vi "LDP Control.vi"() -> ()   [LabVIEW 2017]
uses:
  <instrlib>/tio-labview/TIO Library/TIO Stream Open.vi
  <instrlib>/tio-labview/TIO Library/TIO RPC Send REQuest.vi
  <vilib>/Utility/error.llb/Clear Errors.vi
  <instrlib>/tio-labview/TIO Library/TIO RPC Parse Reply.vi
  <instrlib>/tio-labview/TIO Library/TIO RPC Parse Reply Error.vi
  <instrlib>/tio-labview/TIO Library/TIO Data Stream Parse timebase Info.vi
  <instrlib>/tio-labview/TIO Library/TIO Data Stream Parse pstream Info.vi
  <instrlib>/tio-labview/TIO Library/TIO Data Stream Parse dstream Info.vi
  <vilib>/Utility/High Resolution Relative Seconds.vi
  <instrlib>/tio-labview/TIO Library/TIO Serial Port Name Search.vi
  <instrlib>/tio-labview/TIO Library/TIO Stream Write.vi
  <instrlib>/tio-labview/TIO Library/TIO RPC Form Request.vi
  <instrlib>/tio-labview/TIO Library/TIO SLIP Serial Write.vi
  <instrlib>/tio-labview/TIO Library/TIO Form Packet.vi
  <instrlib>/tio-labview/TIO Library/TIO SLIP Encode.vi
  <instrlib>/tio-labview/TIO Library/TIO Serial Checksum CRC32.vi
  <vilib>/Utility/tcp.llb/UDP Multicast Open.vi
  <vilib>/Utility/tcp.llb/UDP Multicast Read-Write Open.vi
  <instrlib>/tio-labview/TIO Library/TIO Serial Port Discovery.vi
  <vilib>/Instr/_visa.llb/VISA Configure Serial Port (Instr).vi
  <instrlib>/tio-labview/TIO Library/TIO RPC Blocking.vi
  <instrlib>/tio-labview/TIO Library/TIO Stream Read Non-blocking.vi
  <instrlib>/tio-labview/TIO Library/TIO RPC Send Heartbeat.vi
panel:
  in  "Pulse rate":dbl[unit] format="%#_4g"
  in  "Cal Temperature":dbl[unit] format="%#_4g"
  in  "Laser Voltage":dbl[unit] format="%#_4g"
  out "Resistance":dbl[unit] format="%#_4g"
  in  "Calibrate R0":bool
  in  "TEC Enable":bool
  out "Temperature":dbl[unit] format="%#_4g"
  in  "Temperature Set":dbl[unit] format="%#_4g"
  in  "URL":refnum<visa-resource-name>="tcp://localhost"
  out "ID":string
  in  "Quit":bool
  in  "Duration":dbl[unit]=100.0
  in  "Reset":bool
  out "Temperature Graph":T1(graph)
  # "Pulsed Laser"
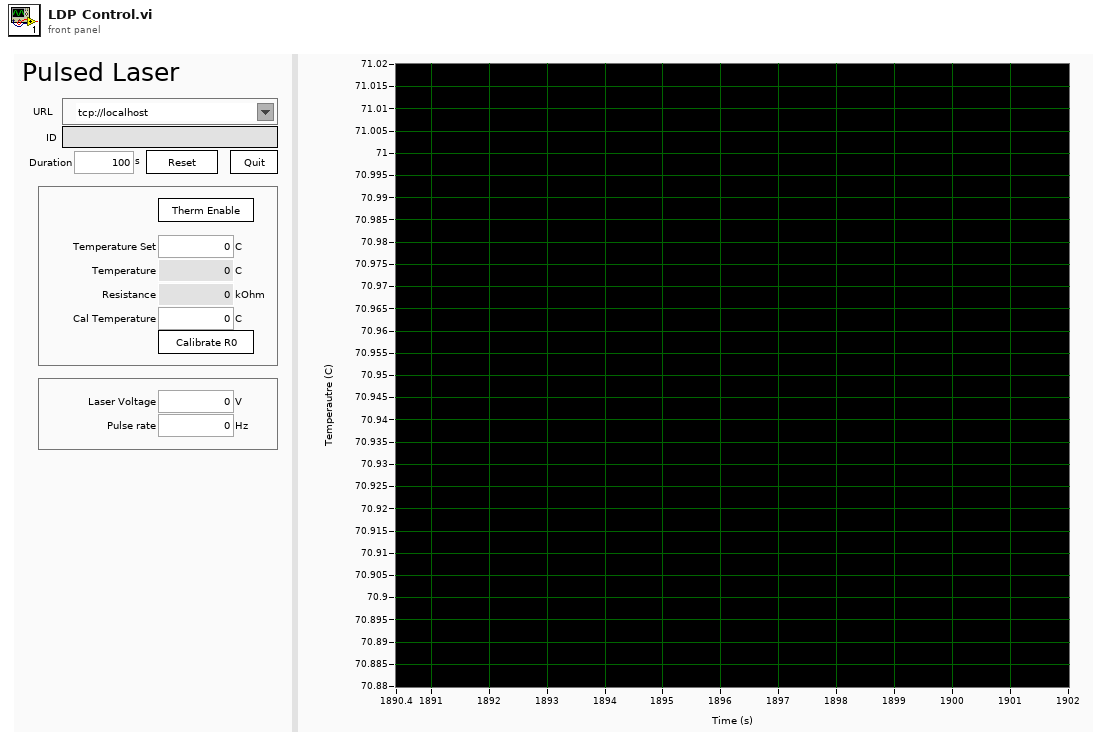
[diagram p1: front panel]
types:
  T1 = cluster{"start":dbl, "dt":dbl, "Timeseries":dbl[]}
  T2 = cluster{"TS Connection":cluster{"Type":enum16{"Serial", "TCP", "UDP", "mUDP"}, "URL":refnum<visa-resource-name>, "TO":u32, "Addr":u32, "Port":i32, "TCP":refnum<k5>, "UDP":refnum<k16>, "Route":string}, "REQ":refnum<queue>, "REP":refnum<queue>}
  T3 = cluster{"Awaiting REP":bool, "REQ ID":u32, "streams in":cluster{"id":u16, "timebase id":u16, "period":u32, "offset":u32, "sample number":u64, "total components":u16, "flags":u16, "components":cluster{"source id":u16, "flags":u16, "period":u32, "offset":u32}[]}[], "sources":cluster{"id":u16, "timebase_id":u16, "period":u32, "offset":u32, "fmt":i32, "flags":u16, "channels":u16, "type":u8, "name":string, "column names":string[], "title":string, "units":string}[], "timebases":cluster{"id":u16, "source":u8, "epoch":u8, "start time":u64, "period numerator (µs)":u32, "period denominator (µs)":u32, "flags":u32, "stability":sgl, "source id":string}[]}
  T4 = cluster{"stream ID":u16, "Sample Number":u32, "Raw Data":string}
  T5 = cluster{"TC Connection":cluster{"Type":enum16{"Serial", "TCP", "UDP", "mUDP"}, "URL":refnum<visa-resource-name>, "TO":u32, "Addr":u32, "Port":i32, "TCP":refnum<k5>, "UDP":refnum<k16>, "Route":string}, "REQ":refnum<queue>, "REP":refnum<queue>}
  T6 = cluster{"Name":string, "Waveform":cluster{"start":dbl, "dt":dbl, "Timeseries":dbl[][]}}[]
  T7 = cluster{"start":dbl, "dt":dbl, "Timeseries":dbl[][]}
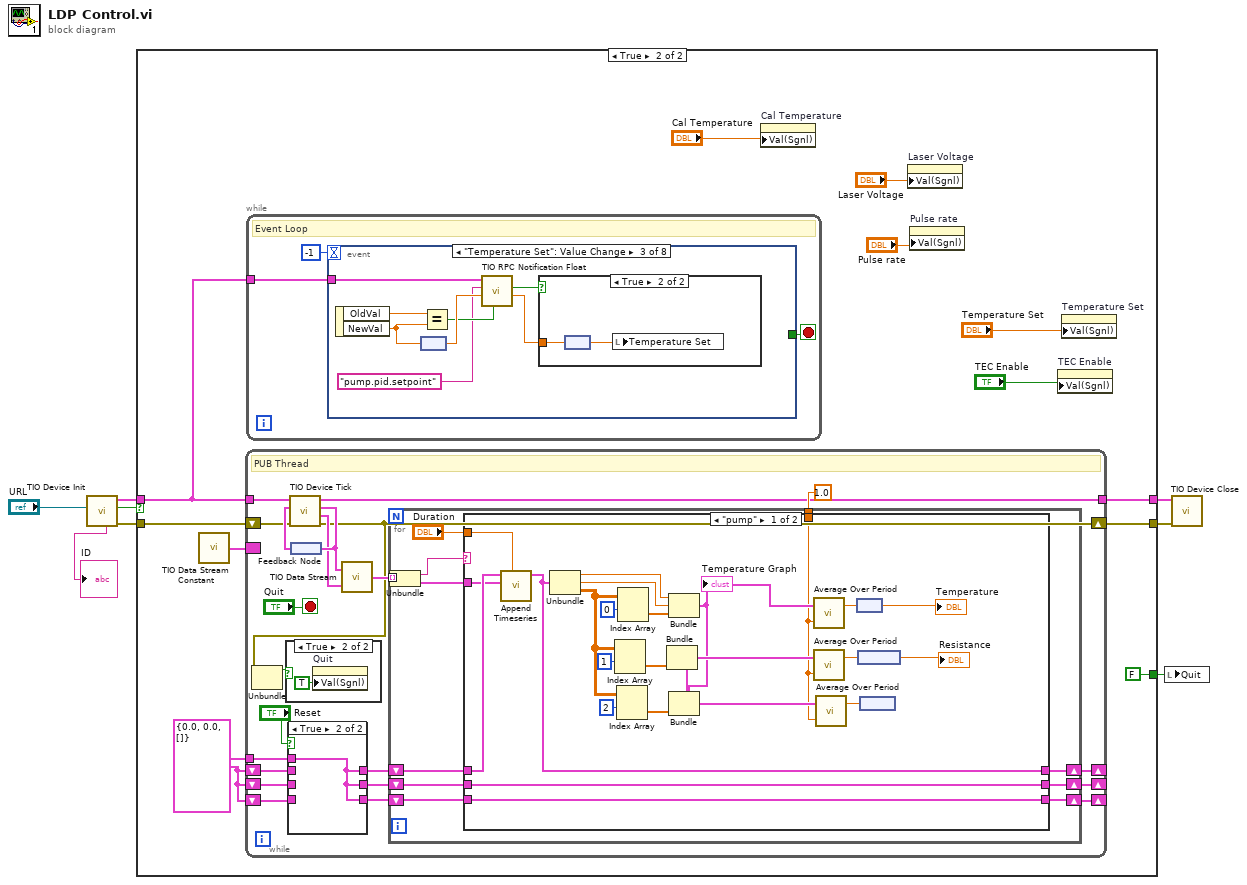
[diagram p0: block diagram]
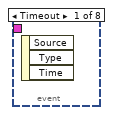
[diagram p6: hidden frame]
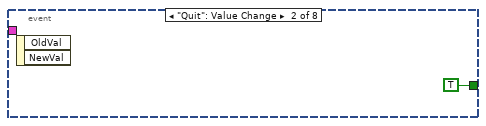
[diagram p7: hidden frame]
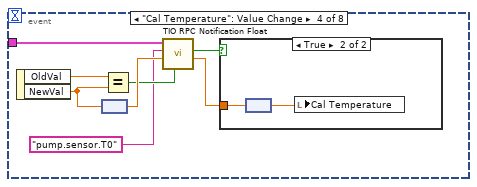
[diagram p9: hidden frame]
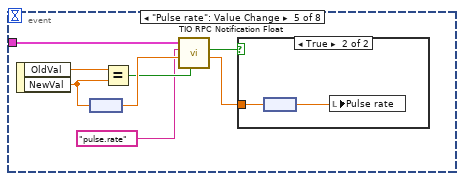
[diagram p11: hidden frame]
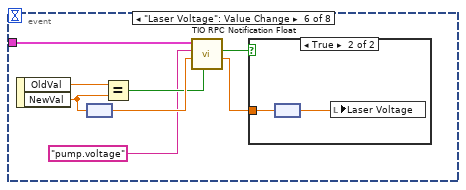
[diagram p13: hidden frame]
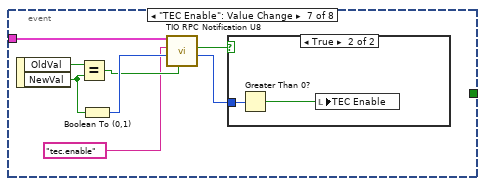
[diagram p15: hidden frame]
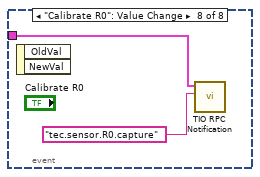
[diagram p17: hidden frame]
diagram:
  n1 = call <instrlib>:"TIO Device Init.vi"("URL"="URL") -> ("error out"=w5:errorcluster, 2:"ID Verified"=w6:bool, "TIO"=w7:T2, 4:"ID Verified"=→"ID":string)  [unwired: 6 in, 1 out]
  n2 = case shown="True" w6 {
    tunnel: w7 -> [w10 w17]
    tunnel: w5 -> [w9 w18]
    tunnel: [_ FALSE ("Quit")] -> w4
    tunnel: [w9 w13] -> w3
    tunnel: [w10 w12] -> w2
    frame False {
    }
    frame True {
      w14 = cluster{dbl, dbl, dbl[][]} {0.0, 0.0, []} ("Waveform Timeseries")
      n3 = call <instrlib>:"TIO Data Stream Constant.vi"() -> ("TIO State"=w19:T3)
      n4 = while {
        shift-right: [w44] -> _
        shift-left: w14 -> [w34]
        border: w19 -> [_]
        tunnel: w17 -> [w40]
        tunnel: w14 -> [w33]
        shift-right: [w31] -> _
        shift-left: w14 -> [w30]
        shift-right: [w27] -> _
        shift-left: w14 -> [w28]
        tunnel: [w24] -> w12
        shift-right: [w23] -> w13
        shift-left: w18 -> [w39]
        stop <- "Quit" stop-if-true
        # "PUB Thread"
        n5 = case shown="True" "Reset" {
          tunnel: [w48 w49] -> w35
          tunnel: w34 -> [w48 _]
          tunnel: w33 -> [_ w49]
          tunnel: [w47 w49] -> w32
          tunnel: w30 -> [w47 _]
          tunnel: w28 -> [w46 _]
          tunnel: [w46 w49] -> w29
          frame False {
          }
          frame True {
          }
        }
        n6 = feedback #1() -> (w43:T3)
        n7 = call <instrlib>:"TIO Device Tick.vi"("Error in"=w39, "TIO State"=w43, "TIO"=w40) -> ("Error out"=w23:errorcluster, "Data Out"=w41:T4, "TIO State"=w42:T3, "TIO"=w24:T5)  [unwired: 5 in]
        n8 = Unbundle(w23) -> ("status"=w25:bool)  [unwired: 2 out]
        n9 = case shown="True" w25 {
          frame False {
          }
          frame True {
            n10 = property on="Quit" class="Bool (strict)"("Val(Sgnl)"=TRUE ("Value (Signaling)")) -> ()  [unwired: 2 in, 2 out]
          }
        }
        n11 = feedback-in #1(w42) -> ()
        n12 = call <instrlib>:"TIO Data Stream.vi"("Raw Data"=w41, "TIO State"=w42) -> ("Data Out"=w38:T6)
        n13 = for {
          shift-right: [w59] -> w44
          shift-left: w35 -> [w58]
          tunnel: w38 -> [w57] mode=indexing
          shift-right: [w53] -> w31
          shift-left: w32 -> [w54]
          shift-right: [w51] -> w27
          shift-left: w29 -> [w52]
          tunnel: dbl[unit] 1.0 ("Period") -> [w50]
          n14 = Unbundle(w57) -> ("Name"=w55:string, "Waveform"=w56:T7)
          n15 = case shown="\"pump\"" w55 {
            tunnel: "Duration" -> [w84 _]
            tunnel: [w82 w87] -> w59
            tunnel: w58 -> [w81 w87]
            tunnel: w56 -> [w64 _]
            tunnel: w54 -> [w63 w86]
            tunnel: [w63 w86] -> w53
            tunnel: [w62 w85] -> w51
            tunnel: w52 -> [w62 w85]
            tunnel: w50 -> [w61 _]
            frame "pump" {
              n16 = call <instrlib>:"Append Timeseries.vi"("Duration"=w84, "In New"=w64, "In Old"=w81) -> ("Appended"=w82:T7)  [unwired: 8 in]
              n17 = Unbundle(w82) -> ("start"=w68:dbl, "dt"=w67:dbl, "Timeseries"=w69:dbl[][])
              n18 = Index Array(array=w69, index (row)=1 ("disabled index (col)")) -> (element=w71:dbl[])  [unwired: 1 in]
              n19 = Index Array(array=w69, index (row)=2 ("disabled index (col)")) -> (element=w76:dbl[])  [unwired: 1 in]
              n20 = Index Array(array=w69, index (row)=0 ("disabled index (col)")) -> (element=w80:dbl[])  [unwired: 1 in]
              n21 = Bundle("start"=w68, "dt"=w67, "Timeseries"=w80) -> (w65:T1)  [unwired: 1 in]
              "Temperature Graph" <- w65
              n22 = Bundle(cluster=w65, "Timeseries"=w71) -> (w72:T1)  [unwired: 2 in]
              n23 = Bundle(cluster=w65, "Timeseries"=w76) -> (w75:T1)  [unwired: 2 in]
              n24 = call <instrlib>:"Average Over Period.vi"("Average Period"=w61, "Waveform"=w65) -> ("Average"=w79:dbl)  [unwired: 1 in]
              n25 = call <instrlib>:"Average Over Period.vi"("Average Period"=w61, "Waveform"=w72) -> ("Average"=w73:dbl)  [unwired: 1 in]
              n26 = call <instrlib>:"Average Over Period.vi"("Average Period"=w61, "Waveform"=w75) -> ("Average"=w74:dbl)  [unwired: 1 in]
              n27 = node(w79) -> (→"Temperature":dbl[unit])
              n28 = node(w73) -> (→"Resistance":dbl[unit])
              n29 = node(w74) -> ()  [unwired: 1 out]
            }
            frame Default {
            }
          }
        }
      }
      n30 = while {
        tunnel: w17 -> [w89]
        stop <- w88 stop-if-true
        # "Event Loop"
        n31 = event shown="[2] \"Temperature Set\": Value Change" {
          selector: _ -> [_ _ _ _ _ _ _ _]
          dyn-events: _ -> [_ _ _ _ _ _ _ _]
          timeout: -1 -> [_ _ _ _ _ _ _ _]
          tunnel: w89 -> [_ _ w94 w104 w114 w124 w134 w143]
          tunnel: [_ TRUE ("Quit") _ _ _ _ _ _] -> w88
          event Timeout {
            n32 = event-data() -> ()  [unwired: 1 in, 3 out]
          }
          event "Quit": Value Change {
            n33 = event-data() -> ()  [unwired: 1 in, 2 out]
          }
          event "Temperature Set": Value Change {
            n34 = event-data() -> ("OldVal"=w99:dbl[unit], "NewVal"=w95:dbl[unit])  [unwired: 1 in]
            n35 = node(w95) -> (w98:dbl)
            n36 = Equal?(x=w99, y=w95) -> (x = y?=w93:bool)
            n37 = call <instrlib>:"TIO RPC Notification Float.vi"("Read"=w93, "Set value"=w98, "Topic"="pump.pid.setpoint" ("String"), "TIO"=w94) -> ("Get value (default if error)"=w96:sgl, "Response"=w97:bool)  [unwired: 4 in, 1 out]
            n38 = case shown="True" w97 {
              tunnel: w96 -> [_ w101]
              frame False {
              }
              frame True {
                n39 = node(w101) -> (w100:sgl[unit])
                n40 = local write "Temperature Set"(w100) -> ()
              }
            }
          }
          event "Cal Temperature": Value Change {
            n41 = event-data() -> ("OldVal"=w109:dbl[unit], "NewVal"=w105:dbl[unit])  [unwired: 1 in]
            n42 = node(w105) -> (w108:dbl)
            n43 = Equal?(x=w109, y=w105) -> (x = y?=w103:bool)
            n44 = call <instrlib>:"TIO RPC Notification Float.vi"("Read"=w103, "Set value"=w108, "Topic"="pump.sensor.T0" ("String"), "TIO"=w104) -> ("Get value (default if error)"=w106:sgl, "Response"=w107:bool)  [unwired: 4 in, 1 out]
            n45 = case shown="True" w107 {
              tunnel: w106 -> [_ w111]
              frame False {
              }
              frame True {
                n46 = node(w111) -> (w110:sgl[unit])
                n47 = local write "Cal Temperature"(w110) -> ()
              }
            }
          }
          event "Pulse rate": Value Change {
            n48 = event-data() -> ("OldVal"=w119:dbl[unit], "NewVal"=w115:dbl[unit])  [unwired: 1 in]
            n49 = node(w115) -> (w118:dbl)
            n50 = Equal?(x=w119, y=w115) -> (x = y?=w113:bool)
            n51 = call <instrlib>:"TIO RPC Notification Float.vi"("Read"=w113, "Set value"=w118, "Topic"="pulse.rate" ("String"), "TIO"=w114) -> ("Get value (default if error)"=w116:sgl, "Response"=w117:bool)  [unwired: 4 in, 1 out]
            n52 = case shown="True" w117 {
              tunnel: w116 -> [_ w121]
              frame False {
              }
              frame True {
                n53 = node(w121) -> (w120:sgl[unit])
                n54 = local write "Pulse rate"(w120) -> ()
              }
            }
          }
          event "Laser Voltage": Value Change {
            n55 = event-data() -> ("OldVal"=w129:dbl[unit], "NewVal"=w125:dbl[unit])  [unwired: 1 in]
            n56 = node(w125) -> (w128:dbl)
            n57 = Equal?(x=w129, y=w125) -> (x = y?=w123:bool)
            n58 = call <instrlib>:"TIO RPC Notification Float.vi"("Read"=w123, "Set value"=w128, "Topic"="pump.voltage" ("String"), "TIO"=w124) -> ("Get value (default if error)"=w126:sgl, "Response"=w127:bool)  [unwired: 4 in, 1 out]
            n59 = case shown="True" w127 {
              tunnel: w126 -> [_ w131]
              frame False {
              }
              frame True {
                n60 = node(w131) -> (w130:sgl[unit])
                n61 = local write "Laser Voltage"(w130) -> ()
              }
            }
          }
          event "TEC Enable": Value Change {
            n62 = event-data() -> ("OldVal"=w139:bool, "NewVal"=w135:bool)  [unwired: 1 in]
            n63 = Equal?(x=w139, y=w135) -> (x = y?=w133:bool)
            n64 = Boolean To (0,1)(Boolean=w135) -> (0, 1=w138:i16)
            n65 = call <instrlib>:"TIO RPC Notification U8.vi"("Read"=w133, "U8"=w138, "Topic"="tec.enable" ("String"), "TIO"=w134) -> ("U8"=w136:u8, "Response"=w137:bool)  [unwired: 4 in, 1 out]
            n66 = case shown="True" w137 {
              tunnel: w136 -> [_ w141]
              frame False {
              }
              frame True {
                n67 = Greater Than 0?(x=w141) -> (x > 0?=w140:bool)
                n68 = local write "TEC Enable"(w140) -> ()
              }
            }
          }
          event "Calibrate R0": Value Change {
            n69 = event-data() -> ()  [unwired: 1 in, 2 out]
            n70 = call <instrlib>:"TIO RPC Notification.vi"("Topic"="tec.sensor.R0.capture" ("String"), "TIO"=w143) -> ()  [unwired: 6 in, 3 out]
          }
        }
      }
      n71 = property on="Cal Temperature" class="DigNum (strict)"("Val(Sgnl)"="Cal Temperature") -> ()  [unwired: 2 in, 2 out]
      n72 = property on="Laser Voltage" class="DigNum (strict)"("Val(Sgnl)"="Laser Voltage") -> ()  [unwired: 2 in, 2 out]
      n73 = property on="Pulse rate" class="DigNum (strict)"("Val(Sgnl)"="Pulse rate") -> ()  [unwired: 2 in, 2 out]
      n74 = property on="TEC Enable" class="Bool (strict)"("Val(Sgnl)"="TEC Enable") -> ()  [unwired: 2 in, 2 out]
      n75 = property on="Temperature Set" class="DigNum (strict)"("Val(Sgnl)"="Temperature Set") -> ()  [unwired: 2 in, 2 out]
    }
  }
  n76 = local write "Quit"(w4) -> ()
  n77 = call <instrlib>:"TIO Device Close.vi"("Error in"=w3, "TIO"=w2) -> ()  [unwired: 10 in]
